vi "LoadPatientDateInfo_ArmPressure-Kamronn-Medtech.vi"(8 "error in":errorcluster, 11 "File path":path) -> (0 "error out":errorcluster, 2 "Armpressure Left":T1(array[cluster]), 3 "Armpressure Right":T1(array[cluster]))   [LabVIEW 2013, in "main.lvlib"]
uses:
  main.lvlib
  Controls/date_specific_info.ctl
  Globals/DataPathGlobalVariable.vi
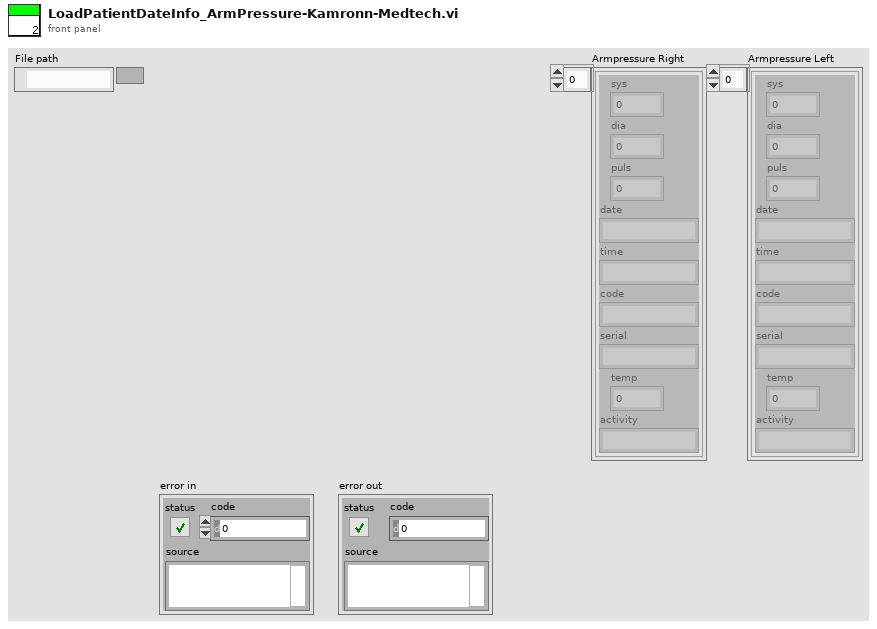
[diagram p1: front panel]
types:
  T1 = cluster{"sys":dbl, "dia":dbl, "puls":dbl, "date":string, "time":string, "code":string, "serial":string, "temp":dbl, "activity":string}[]
  T2 = typedef "main.lvlib/date_specific_info.ctl" = cluster{"profile":cluster{"id":string, "name":string, "operator":string, "doctor":string, "comment":string}, "hospital":cluster{"name":string, "department":string, "address":string}, "palpation":cluster{"right":string, "left":string}, "Armpressure Right":cluster{"sys":dbl, "dia":dbl, "puls":dbl, "date":string, "time":string, "code":string, "serial":string, "temp":dbl, "activity":string}[], "Armpressure Left":cluster{"sys":dbl, "dia":dbl, "puls":dbl, "date":string, "time":string, "code":string, "serial":string, "temp":dbl, "activity":string}[]}
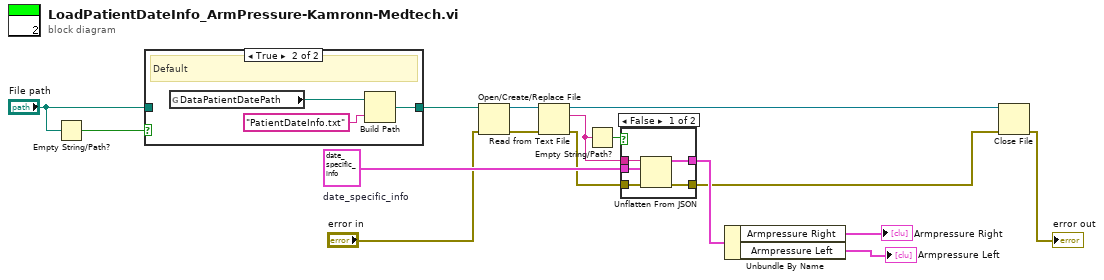
[diagram p0: block diagram]
diagram:
  w16 = T2 {"profile"={"id"="", "name"="", "operator"="", "doctor"="", "comment"=""}, "hospital"={"name"="", "department"="", "address"=""}, "palpation"={"right"="", "left"=""}, "Armpressure Right"=[], "Armpressure Left"=[]}  # date_specific_info
  n1 = Empty String/Path?(string/path="File path") -> (empty?=w2:bool)
  n2 = case shown="True" w2 {
    tunnel: [w17 w18] -> w6
    tunnel: "File path" -> [w17 _]
    frame False {
    }
    frame True {
      # "Default"
      n3 = global read "DataPathGlobalVariable.vi" "DataPatientDatePath"() -> (w20:path)
      n4 = Build Path(base path=w20, name or relative path="PatientDateInfo.txt") -> (appended path=w18:path)
    }
  }
  n5 = Open/Create/Replace File(file path (use dialog)=w6, error in="error in") -> (refnum out=w5:refnum<file>, error out=w4:errorcluster)  [unwired: 4 in, 1 out]
  n6 = Read from Text File(file (use dialog)=w5, error in=w4) -> (refnum out=w12:refnum<file>, text=w8:string, error out=w15:errorcluster)  [unwired: 2 in, 1 out]
  n7 = Empty String/Path?(string/path=w8) -> (empty?=w7:bool)
  n8 = case shown="False" w7 {
    tunnel: w16 -> [w25 w26]
    tunnel: w15 -> [w24 w27]
    tunnel: [w23 w26] -> w13
    tunnel: [w22 w27] -> w11
    tunnel: w8 -> [w21 _]
    frame False {
      n9 = Unflatten From JSON(JSON string=w21, type and defaults=w25, error in (no error)=w24) -> (value=w23:T2, error out=w22:errorcluster)  [unwired: 4 in]
    }
    frame True {
    }
  }
  n10 = Unbundle By Name(w13) -> ("Armpressure Right"=→"Armpressure Right":T1, "Armpressure Left"=→"Armpressure Left":T1)
  n11 = Close File(refnum=w12, error in=w11) -> (error out=→"error out":errorcluster)  [unwired: 1 out]
